vi "Demo.vi"() -> ()   [LabVIEW 2010]
doc: "本VI是为《我和LabVIEW》一书编写的示例。\n关于本书的介绍请参考网页：\nhttp://ruanqizhen.spaces.live.com/blog/cns!5852D4F797C53FB6!4310.entry"
uses:
  Twinkle Button.xctl
panel:
  in  "Twinkle Button":enum16{"Red", "Green", "Blue"}(xcontrol)
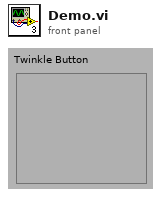
[diagram p1: front panel]
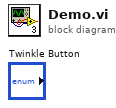
[diagram p0: block diagram]
diagram:
